vi "Write Stop.vi"(8 "error in (no error)":errorcluster, 10 "Stop":bool, 11 "Model Driver in":refnum<class "Model Driver.lvclass">) -> (0 "error out":errorcluster, 3 "Model Driver out":refnum<class "Model Driver.lvclass">)   [LabVIEW 2023, in "Model Driver.lvclass"]
uses:
  Model Driver.lvclass
  Model Driver.lvclass/Model Driver.ctl
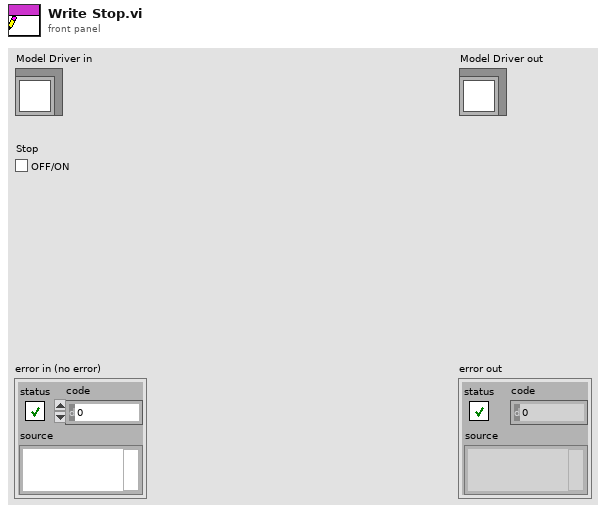
[diagram p1: front panel]
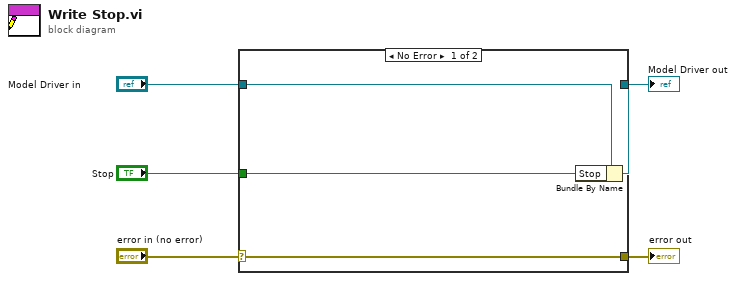
[diagram p0: block diagram]
diagram:
  n1 = case shown="No Error" "error in (no error)" {
    selector: "error in (no error)" -> [w9 w10]
    tunnel: [w9 w10] -> w4
    tunnel: [w7 w11] -> w2
    tunnel: "Model Driver in" -> [w8 w11]
    tunnel: "Stop" -> [w6 _]
    frame No Error {
      n2 = Bundle By Name(cluster=w8, "Stop"=w6) -> (w7:refnum<class "Model Driver.lvclass">)
    }
    frame Error {
    }
  }
  "error out" <- w4
  "Model Driver out" <- w2
